vi "U8ToString.vi"(8 "error in (no error)":errorcluster, 11 "ArrayU8 out":u8[](array[numeric]) format="%02x") -> (0 "error out":errorcluster, 3 "HEX text in":string)   [LabVIEW 2011, in "i3-external-encryption.lvlib"]
doc: "This VI converts an array of U8 into an ASCII HEX string (ascii values 0-f)."
uses:
  i3-external-encryption.lvlib
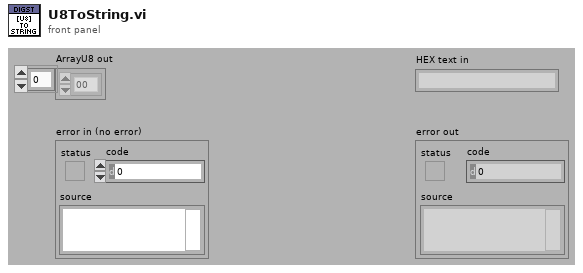
[diagram p1: front panel]
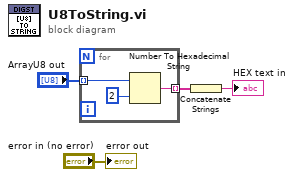
[diagram p0: block diagram]
diagram:
  n1 = for {
    tunnel: [w5] -> w3 mode=indexing
    tunnel: "ArrayU8 out" -> [w6] mode=indexing
    n2 = Number To Hexadecimal String(1:i16 2 ("width (-)"), 2:w6) -> (0:w5:string)
  }
  n3 = Concatenate Strings(w3) -> (→"HEX text in":string)
  "error out" <- "error in (no error)"
